vi "update.labels.vi"(8 "error in (no error)":errorcluster, 10 "Labels":string[](array[string]), 11 "event in":refnum<class "event.lvclass">) -> (0 "error out":errorcluster, 3 "event out":refnum<class "event.lvclass">)   [LabVIEW 2020, in "event.lvclass"]
uses:
  event.lvclass
  event.lvclass/event.ctl
  Nominal Client/Nominal Client.lvclass/Nominal Client.ctl
  Nominal Client/error.vi
  Nominal Client/trace.payload_sent.vi
  Nominal Client/trace.payload_received.vi
  Nominal Client/create.authorization_header.vi
  Nominal Client/error.vi/859f8e04-e495-489b-b5b4-7ac163f56130.vi
  Nominal Client/trace.calling_method.vi
  <vilib>/JDP Science/JDP Science Common Utilities/Trim Whitespace__JDP.vi
  <vilib>/AdvancedString/1D String Array to Delimited String.vi
  Nominal Client/api_token.get.vi
  <vilib>/Utility/libraryn.llb/Get File Extension.vi
  Nominal Client/log_file.write.vi
  <vilib>/JDP Science/JSONtext/Get all Object Items.vi
  <vilib>/Utility/error.llb/Error Cluster From Error Code.vi
  <vilib>/JDP Science/JSONtext/JSON text to Variant.vi
  <vilib>/JDP Science/JSONtext/LVClass Serializer/JSONtext LVClass Serializer.lvclass
  <vilib>/addons/_JKI.lib/REST Client/classes/Response Headers/Response Headers.lvclass
  <vilib>/addons/_JKI.lib/REST Client/classes/REST Client/REST Client.lvclass
  Nominal Client/Nominal Client.lvclass
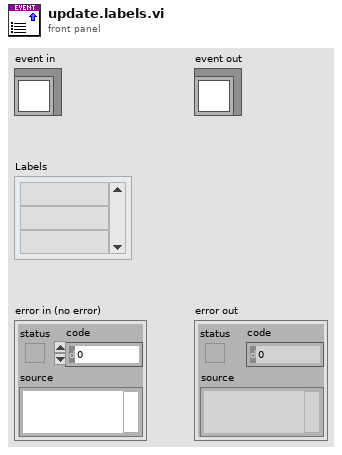
[diagram p1: front panel]
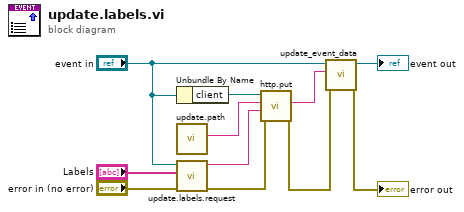
[diagram p0: block diagram]
diagram:
  n1 = Unbundle By Name("event in") -> ("client"=w11:refnum<class "Nominal Client.lvclass">)
  n2 = call "update.path.vi"() -> ("path"=w10:string)  [unwired: 11 in]
  n3 = call "update.labels.request.vi"("error in"="error in (no error)", "Labels"="Labels", "event"="event in") -> ("error out"=w9:errorcluster, "request"=w7:string)  [unwired: 7 in]
  n4 = call "http.put.vi"("error in"=w9, "Body"=w7, "Path"=w10, "Nominal Client in"=w11) -> ("error out"=w3:errorcluster, "Response"=w6:string)  [unwired: 4 in, 2 out]
  n5 = call "update_event_data.vi"("error in"=w3, "JSON"=w6, "event in"="event in") -> ("error out"=→"error out":errorcluster, "event out"=→"event out":refnum<class "event.lvclass">)  [unwired: 7 in]
